vi "Destroy.vi"(0 "LV MDI in":refnum<class "LV MDI.lvclass">, 11 "error in (no error)":errorcluster) -> (4 "LV MDI out":refnum<class "LV MDI.lvclass">, 15 "error out":errorcluster)   [LabVIEW 2016, in "LV MDI.lvclass"]
doc: "Destroy reference of MDI Panel."
uses:
  LV MDI.lvclass
  LV MDI.lvclass/LV MDI.ctl
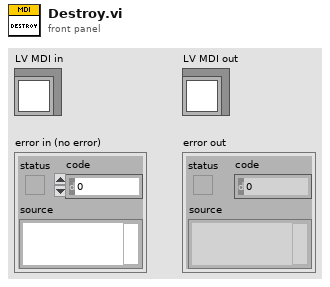
[diagram p1: front panel]
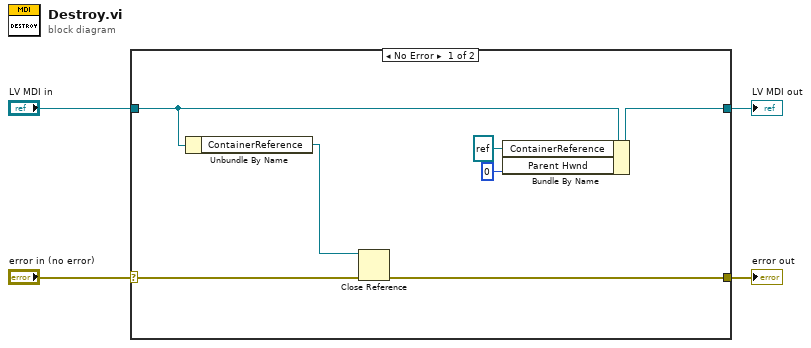
[diagram p0: block diagram]
diagram:
  n1 = case shown="No Error" "error in (no error)" {
    selector: "error in (no error)" -> [w11 w13]
    tunnel: [w10 w13] -> w3
    tunnel: [w7 w12] -> w1
    tunnel: "LV MDI in" -> [w8 w12]
    frame No Error {
      n2 = Unbundle By Name(w8) -> ("ContainerReference"=w9:refnum<k24>)
      n3 = Close Reference(reference=w9, error in (no error)=w11) -> (error out=w10:errorcluster)
      n4 = Bundle By Name(cluster=w8, "ContainerReference"=refnum<k24> refnum ("Container reference"), "Parent Hwnd"=0 ("hWnd")) -> (w7:refnum<class "LV MDI.lvclass">)
    }
    frame Error {
    }
  }
  "error out" <- w3
  "LV MDI out" <- w1
